vi "receive status update.vi"(8 "Message handler data in":T2, 10 "Data":variant, 11 "RT Queues":T1) -> (0 "Message handler data out":T2)   [LabVIEW 2018]
uses:
  Type Defs/Message loop data.ctl
  Type Defs/FPGA reference.ctl
  Type Defs/RT Status.ctl
  Type Defs/Queues cluster.ctl
  ICL-LabVIEW_General/Message Scheduler/message scheduler.lvclass
  Communications loop/create incident - command.vi
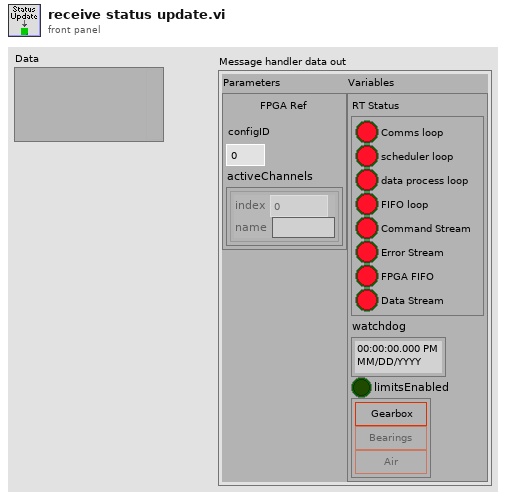
[diagram p1: front panel]
types:
  T1 = typedef "Queues cluster.ctl" = cluster{"RT Message":refnum<queue>, "RT Comms":refnum<queue>, "RT Data":refnum<queue>, "RT FIFO":refnum<queue>, "message scheduler":refnum<class "message scheduler.lvclass">}
  T2 = typedef "Message loop data.ctl" = cluster{"Parameters":cluster{"FPGA Ref":T3, "configID":u32, "activeChannels":cluster{"index":u16, "name":string}[]}, "Variables":cluster{"RT Status":T4, "watchdog":timestamp, "limitsEnabled":bool, "Interlocks":cluster{"gearboxOil":bool, "bearingOil":bool, "gearboxAir":bool}}}
  T3 = typedef "FPGA reference.ctl" = refnum<k20>
  T4 = typedef "RT Status.ctl" = cluster{"Comms loop":bool, "scheduler loop":bool, "data process loop":bool, "FIFO loop":bool, "Command Stream":bool, "Error Stream":bool, "FPGA FIFO":bool, "Data Stream":bool}
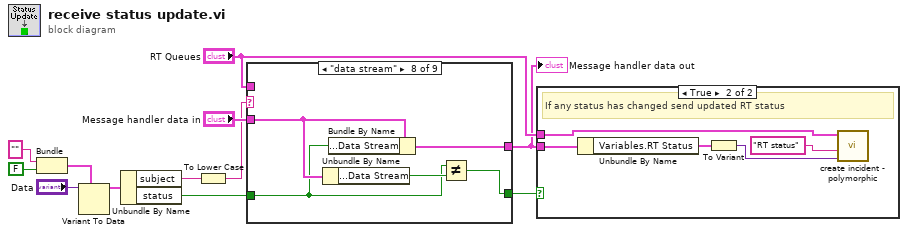
[diagram p0: block diagram]
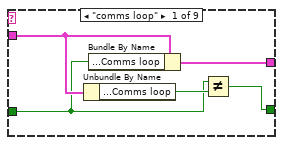
[diagram p3: hidden frame]
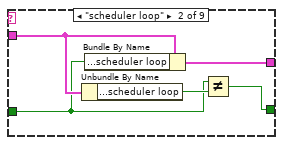
[diagram p4: hidden frame]
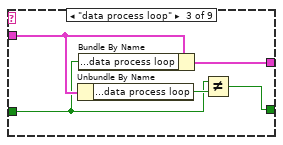
[diagram p5: hidden frame]
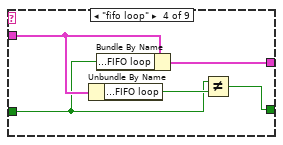
[diagram p6: hidden frame]
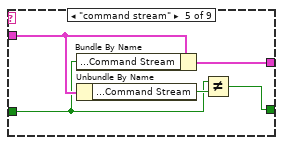
[diagram p7: hidden frame]
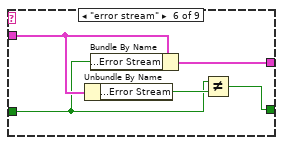
[diagram p8: hidden frame]
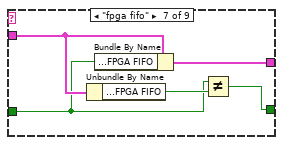
[diagram p9: hidden frame]
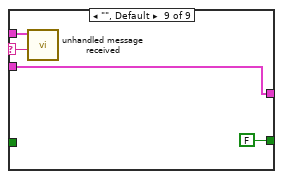
[diagram p10: hidden frame]
diagram:
  n1 = Bundle("subject"="", "status"=FALSE) -> (w8:cluster{"subject":string, "status":bool})  [unwired: 1 in]
  n2 = Variant To Data(type=w8, Variant="Data") -> (data=w7:cluster{"subject":string, "status":bool})  [unwired: 1 in, 1 out]
  n3 = Unbundle By Name(w7) -> ("subject"=w6:string, "status"=w5:bool)
  n4 = To Lower Case(string=w6) -> (all lower case string=w4:string)
  n5 = case shown="\"data stream\"" w4 {
    selector: w4 -> [_ _ _ _ _ _ _ _ w53]
    tunnel: [w17 w22 w27 w32 w37 w42 w47 w52 w56] -> w2
    tunnel: "Message handler data in" -> [w16 w21 w26 w31 w36 w41 w46 w51 w56]
    tunnel: w5 -> [w14 w19 w24 w29 w33 w39 w44 w49 _]
    tunnel: [w13 w18 w23 w28 w34 w38 w43 w48 FALSE] -> w1
    tunnel: "RT Queues" -> [_ _ _ _ _ _ _ _ w54]
    frame "comms loop" {
      n6 = Unbundle By Name(w16) -> ("Variables.RT Status.Comms loop"=w15:bool)
      n7 = Bundle By Name(cluster=w16, "Variables.RT Status.Comms loop"=w14) -> (w17:T2)
      n8 = Not Equal?(x=w14, y=w15) -> (x != y?=w13:bool)
    }
    frame "scheduler loop" {
      n9 = Unbundle By Name(w21) -> ("Variables.RT Status.scheduler loop"=w20:bool)
      n10 = Bundle By Name(cluster=w21, "Variables.RT Status.scheduler loop"=w19) -> (w22:T2)
      n11 = Not Equal?(x=w19, y=w20) -> (x != y?=w18:bool)
    }
    frame "data process loop" {
      n12 = Unbundle By Name(w26) -> ("Variables.RT Status.data process loop"=w25:bool)
      n13 = Bundle By Name(cluster=w26, "Variables.RT Status.data process loop"=w24) -> (w27:T2)
      n14 = Not Equal?(x=w24, y=w25) -> (x != y?=w23:bool)
    }
    frame "fifo loop" {
      n15 = Unbundle By Name(w31) -> ("Variables.RT Status.FIFO loop"=w30:bool)
      n16 = Bundle By Name(cluster=w31, "Variables.RT Status.FIFO loop"=w29) -> (w32:T2)
      n17 = Not Equal?(x=w29, y=w30) -> (x != y?=w28:bool)
    }
    frame "command stream" {
      n18 = Bundle By Name(cluster=w36, "Variables.RT Status.Command Stream"=w33) -> (w37:T2)
      n19 = Unbundle By Name(w36) -> ("Variables.RT Status.Command Stream"=w35:bool)
      n20 = Not Equal?(x=w33, y=w35) -> (x != y?=w34:bool)
    }
    frame "error stream" {
      n21 = Unbundle By Name(w41) -> ("Variables.RT Status.Error Stream"=w40:bool)
      n22 = Bundle By Name(cluster=w41, "Variables.RT Status.Error Stream"=w39) -> (w42:T2)
      n23 = Not Equal?(x=w39, y=w40) -> (x != y?=w38:bool)
    }
    frame "fpga fifo" {
      n24 = Unbundle By Name(w46) -> ("Variables.RT Status.FPGA FIFO"=w45:bool)
      n25 = Bundle By Name(cluster=w46, "Variables.RT Status.FPGA FIFO"=w44) -> (w47:T2)
      n26 = Not Equal?(x=w44, y=w45) -> (x != y?=w43:bool)
    }
    frame "data stream" {
      n27 = Unbundle By Name(w51) -> ("Variables.RT Status.Data Stream"=w50:bool)
      n28 = Bundle By Name(cluster=w51, "Variables.RT Status.Data Stream"=w49) -> (w52:T2)
      n29 = Not Equal?(x=w49, y=w50) -> (x != y?=w48:bool)
    }
    frame "", Default {
      n30 = call "unhandled message received.vi"("unhandled message"=w53, "RT Queues"=w54) -> ()  [unwired: 10 in]
    }
  }
  "Message handler data out" <- w2
  n31 = case shown="True" w1 {
    tunnel: "RT Queues" -> [_ w59]
    tunnel: w2 -> [_ w61]
    frame False {
    }
    frame True {
      # "If any status has changed send updated RT status"
      n32 = Unbundle By Name(w61) -> ("Variables.RT Status"=w60:T4)
      n33 = To Variant(anything=w60) -> (Variant=w57:variant)
      n34 = call-poly "create incident - polymorphic.vi"("data"=w57, "command"="RT status" ("message"), "RT Queues"=w59) -> ()  [unwired: 9 in]
    }
  }
